vi "save server method.vi"(7 "DS method":T1={"scan rate (Hz)"=100.0, "Channel group array"=[], "Number of groups"=1} {"Number of groups" min=1; "Channel group array"."max voltage" format="%.4f"; "scan rate (Hz)" format="%.2f"}) -> ()   [LabVIEW 2012]
uses:
  DataServer/Dataserver method.ctl
panel:
  # "Hz"
  # "channel identifiers"
  # "max voltage"
  # "port locations"
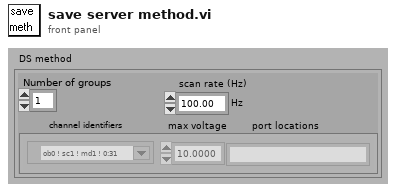
[diagram p1: front panel]
types:
  T1 = typedef "Dataserver method.ctl" = cluster{"scan rate (Hz)":dbl, "Channel group array":cluster{"channels":tag, "max voltage":sgl, "Port locations":string}[], "Number of groups":u8}
  T2 = enum16{"open", "open or create", "create or replace", "create"}
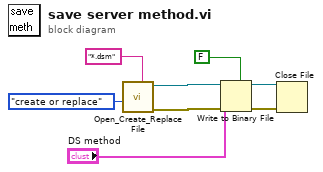
[diagram p0: block diagram]
diagram:
  n1 = call <vilib>:"Open_Create_Replace File.vi"("pattern"="*.dsm", "function (open:0)"=T2."create or replace") -> ("error out"=w7:errorcluster, "refnum"=w6:refnum<file>)  [unwired: 6 in, 2 out]
  n2 = Write to Binary File(file (use dialog)=w6, data="DS method", error in=w7, 5:FALSE ("prepend array or string size? (T)")) -> (refnum out=w3:refnum<file>, error out=w2:errorcluster)  [unwired: 2 in, 1 out]
  n3 = Close File(refnum=w3, error in=w2) -> ()  [unwired: 2 out]
